vi "Consumidor.vi"() -> ()   [LabVIEW 2020]
uses:
  Options.ctl
panel:
  in  "stop":bool
  out "element":string
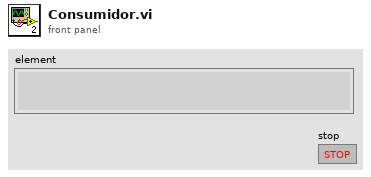
[diagram p1: front panel]
types:
  T1 = typedef "Options.ctl" = enum16{"Create", "Get", "Destroy"}
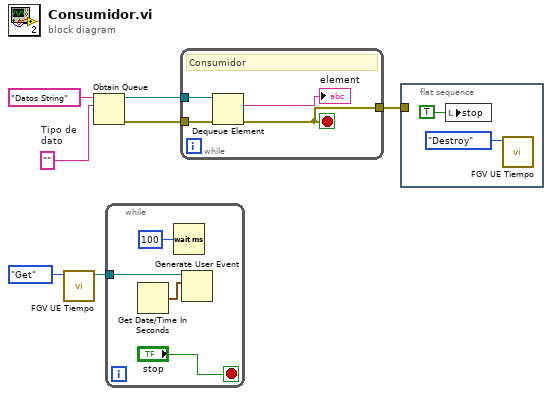
[diagram p0: block diagram]
diagram:
  w7 = ""  # Tipo de dato
  n1 = call "FGV UE Tiempo.vi"("Enum"=Options."Get") -> ("User Event out"=w2:refnum<user-event>)  [unwired: 10 in]
  n2 = Obtain Queue(name (unnamed)="Datos String", element data type=w7) -> (queue out=w5:refnum<queue>, error out=w4:errorcluster)  [unwired: 3 in, 1 out]
  n3 = while {
    tunnel: w2 -> [w11]
    stop <- "stop" stop-if-true
    n4 = Get Date/Time In Seconds() -> (seconds since 1Jan1904=w10:timestamp)
    n5 = Wait (ms)(milliseconds to wait=u32 100) -> ()  [unwired: 1 out]
    n6 = Generate User Event(user event=w11, event data cluster=w10) -> ()  [unwired: 2 in, 2 out]
  }
  n7 = while {
    tunnel: w5 -> [w15]
    tunnel: w4 -> [w13]
    tunnel: [w12] -> w1
    stop <- w12 stop-if-true
    # "Consumidor"
    n8 = Dequeue Element(queue=w15, error in (no error)=w13) -> (element=→"element":string, error out=w12:errorcluster)  [unwired: 1 in, 2 out]
  }
  n9 = flat-sequence {
    tunnel: w1 -> [_]
    frame #0 {
      n10 = local write "stop"(TRUE ("stop")) -> ()
      n11 = call "FGV UE Tiempo.vi"("Enum"=Options."Destroy") -> ()  [unwired: 10 in, 1 out]
    }
  }
